vi "perform_checks_after_FWD_move.vi"(3 "tour_in_progress":T1[](array[typedef]), 4 "no. of squares on chessboard":u8, 5 "chessboard":T2[][](array[typedef])) -> (1 "square_to_move_forward_to":T1, 2 "next action":T4)   [LabVIEW 2020, in "core.lvlib"]
uses:
  core.lvlib
  action.ctl
  core_data/chess_square.ctl
  core_data/neighbour_square.ctl
  core_data/chessboard_index.ctl
  get_chessboard_square.vi
  check_island.vi
  check_head_is_neighbour.vi
  get all unexplored neighbours.vi
  pause (global variable).vi
  core_data/core_data.lvlib
panel:
  # "Development\ncontrols/indicators useful for development and testing, but which are not outputs of the VI"
  # "Input\nInputs to the VI"
  # "Output\nOutputs of the VI"
  # "Description\n\nBlank VI with error handling case. \n\nSummarize the use of this VI in this space."
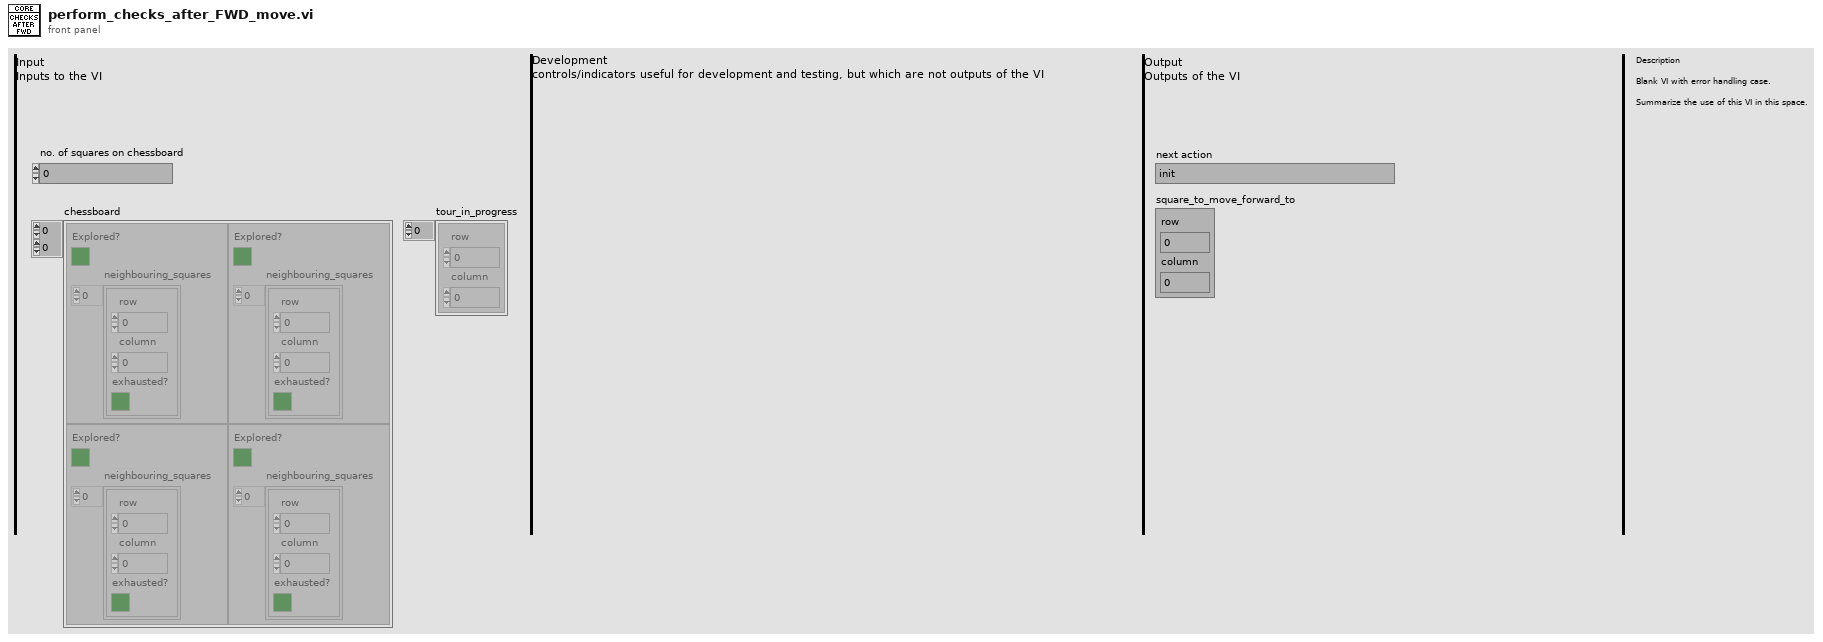
[diagram p1: front panel]
types:
  T1 = typedef "core.lvlib/core_data.lvlib/chessboard_index.ctl" = cluster{"row":u8, "column":u8}
  T2 = typedef "core.lvlib/core_data.lvlib/chess_square.ctl" = cluster{"Explored?":bool, "neighbouring_squares":T3[]}
  T3 = typedef "core.lvlib/core_data.lvlib/neighbour_square.ctl" = cluster{"row":u8, "column":u8, "exhausted?":bool}
  T4 = typedef "core.lvlib/action.ctl" = enum16{"init", "move_forward", "move_backward", "complete_tour", "exit", "be idle (do nothing)"}
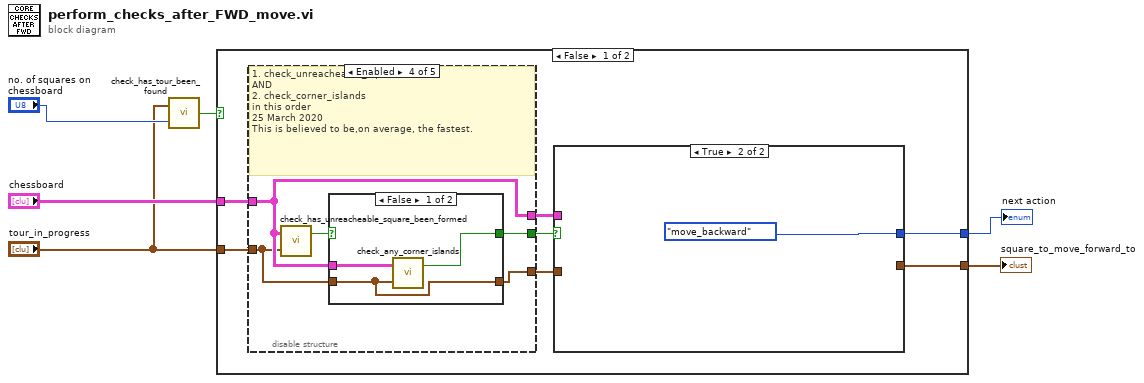
[diagram p0: block diagram]
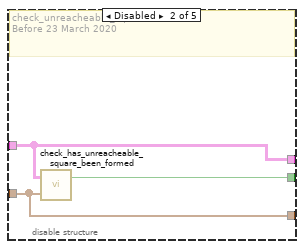
[diagram p3: hidden frame]
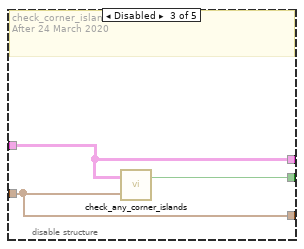
[diagram p4: hidden frame]
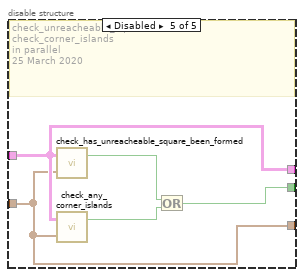
[diagram p6: hidden frame]
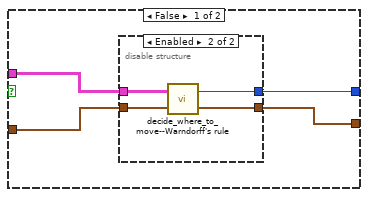
[diagram p7: hidden frame]
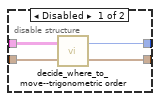
[diagram p8: hidden frame]
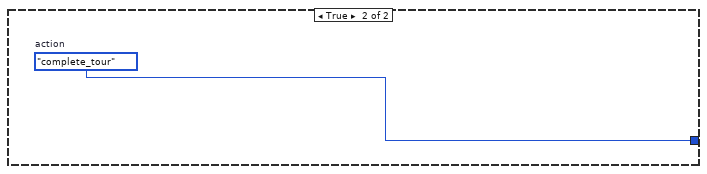
[diagram p9: hidden frame]
diagram:
  n1 = call "check_has_tour_been_found.vi"("no. of squares on chessboard"="no. of squares on chessboard", "tour in progress"="tour_in_progress") -> ("T = complete tour was found"=w6:bool)
  n2 = case shown="False" w6 {
    tunnel: [w13 w50] -> w5
    tunnel: "chessboard" -> [w10 _]
    tunnel: "tour_in_progress" -> [w9 _]
    tunnel: [w7 _] -> w1
    frame False {
      n3 = disable-structure shown="Enabled" {
        disable-tunnel: [_ w18 w21 w26 w35] -> w12
        disable-tunnel: [w15 w17 w20 w24 w36] -> w11
        disable-tunnel: w10 -> [w15 w17 w20 w24 w36]
        disable-tunnel: w9 -> [w14 w16 w19 w23 w32]
        disable-tunnel: [w14 w16 w19 w22 w32] -> w8
        frame Disabled {
          # "skip the \"smart\" checks entirely"
          # "24 Mar 2020 NO CHECKS"
        }
        frame Disabled {
          # "check_unreacheable_square ONLY\nBefore 23 March 2020"
          n4 = call "check_has_unreacheable_square_been_formed.vi"("tour_in_progress"=w16, "chessboard"=w17) -> ("T = unreacheable square found"=w18:bool)  [unwired: 1 out]
        }
        frame Disabled {
          # "check_corner_islands ONLY\nAfter 24 March 2020"
          n5 = call "check_any_corner_islands.vi"("tour_in_progress"=w19, "chessboard"=w20) -> ("T = a corner island was found"=w21:bool)  [unwired: 1 out]
        }
        frame Enabled {
          # "1. check_unreacheable_square\nAND\n2. check_corner_islands\nin this order\n25 March 2020\nThis is believed to be,on average, the fastest."
          n6 = call "check_has_unreacheable_square_been_formed.vi"("tour_in_progress"=w23, "chessboard"=w24) -> ("T = unreacheable square found"=w25:bool)  [unwired: 1 out]
          n7 = case shown="False" w25 {
            selector: w25 -> [_ w31]
            tunnel: [w29 w31] -> w26
            tunnel: w24 -> [w28 _]
            tunnel: w23 -> [w27 w30]
            tunnel: [w27 w30] -> w22
            frame False {
              n8 = call "check_any_corner_islands.vi"("tour_in_progress"=w27, "chessboard"=w28) -> ("T = a corner island was found"=w29:bool)  [unwired: 1 out]
            }
            frame True {
            }
          }
        }
        frame Disabled {
          # "check_unreacheable_square\ncheck_corner_islands\nin parallel\n25 March 2020"
          n9 = call "check_has_unreacheable_square_been_formed.vi"("tour_in_progress"=w32, "chessboard"=w36) -> ("T = unreacheable square found"=w33:bool)  [unwired: 1 out]
          n10 = call "check_any_corner_islands.vi"("tour_in_progress"=w32, "chessboard"=w36) -> ("T = a corner island was found"=w34:bool)  [unwired: 1 out]
          n11 = Or(x=w33, y=w34) -> (x .or. y?=w35:bool)
        }
      }
      n12 = case shown="True" w12 {
        tunnel: [w40 action."move_backward" ("action")] -> w13
        tunnel: w11 -> [w39 _]
        tunnel: w8 -> [w38 _]
        tunnel: [w37 _] -> w7
        frame False {
          n13 = disable-structure shown="Enabled" {
            disable-tunnel: [w44 w46] -> w40
            disable-tunnel: w39 -> [w43 w47]
            disable-tunnel: w38 -> [w42 w48]
            disable-tunnel: [w41 w45] -> w37
            frame Disabled {
              n14 = call "decide_where_to_move--trigonometric order.vi"("tour_in_progress"=w42, "chessboard"=w43) -> ("square_to_move_forward_to"=w41:T1, "action"=w44:T4)
            }
            frame Enabled {
              n15 = call "decide_where_to_move--Warndorff's rule.vi"("tour_in_progress"=w48, "chessboard"=w47) -> ("square_to_move_forward_to"=w45:T1, "action"=w46:T4)
            }
          }
        }
        frame True {
        }
      }
    }
    frame True {
      w50 = action."complete_tour"  # action
    }
  }
  "next action" <- w5
  "square_to_move_forward_to" <- w1
